vi "Multiple Roots.vi"(1 "Polynomial Roots":cdb[](array[numeric]) format="%.2f") -> (0 "multiple roots":bool)   [LabVIEW 2017, in "NI_Gmath.lvlib"]
uses:
  <vilib>/gmath/NI_Gmath.lvlib
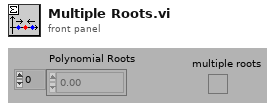
[diagram p1: front panel]
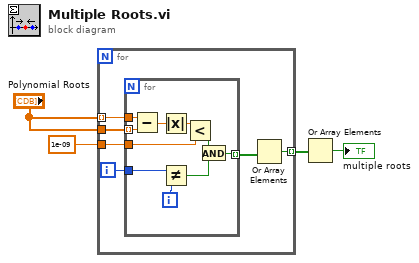
[diagram p0: block diagram]
diagram:
  n1 = for {
    tunnel: "Polynomial Roots" -> [w10] mode=indexing
    tunnel: "Polynomial Roots" -> [w9]
    tunnel: [w6] -> w3 mode=indexing
    tunnel: 1e-09 -> [w5]
    i -> [w8]
    n2 = for {
      tunnel: w10 -> [w14]
      tunnel: w9 -> [w13] mode=indexing
      tunnel: w8 -> [w20]
      tunnel: [w17] -> w7 mode=indexing
      tunnel: w5 -> [w11]
      i -> [w19]
      n3 = Subtract(x=w14, y=w13) -> (x-y=w15:cdb)
      n4 = Absolute Value(x=w15) -> (abs(x)=w12:dbl)
      n5 = Not Equal?(x=w20, y=w19) -> (x != y?=w18:bool)
      n6 = Less?(x=w12, y=w11) -> (x < y?=w16:bool)
      n7 = And(x=w16, y=w18) -> (x .and. y?=w17:bool)
    }
    n8 = Or Array Elements(Boolean array=w7) -> (logical OR=w6:bool)
  }
  n9 = Or Array Elements(Boolean array=w3) -> (logical OR=→"multiple roots":bool)
